vi "face rotate T+.vi"(8 "error in (no error)":errorcluster, 11 "cube in":T1) -> (0 "error out":errorcluster, 3 "cube out":T1)   [LabVIEW 2011]
uses:
  Typedef/cube.ctl
  Typedef/face.ctl
  Typedef/cube rotate direction.ctl
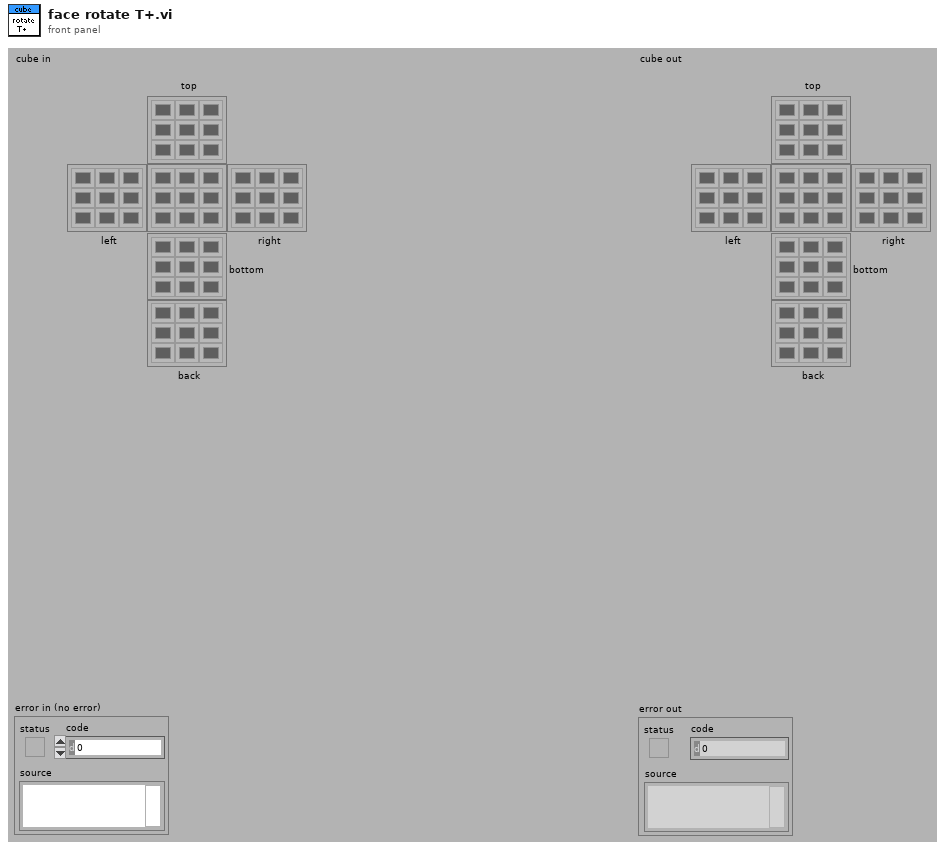
[diagram p1: front panel]
types:
  T1 = typedef "cube.ctl" = cluster{"top":T2, "left":T2, "right":T2, "bottom":T2, "back":T2, "front":T2}
  T2 = typedef "face.ctl" = u32[][]
  T3 = typedef "cube rotate direction.ctl" = enum16{"up", "down", "left", "right"}
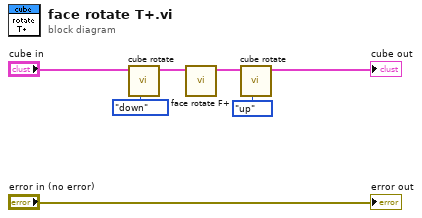
[diagram p0: block diagram]
diagram:
  n1 = call "cube rotate.vi"("cube rotation direction"=cube_rotate_direction."down", "cube in"="cube in") -> ("cube out"=w5:T1)  [unwired: 8 in, 1 out]
  n2 = call "face rotate F+.vi"("cube in"=w5) -> ("cube out"=w3:T1)  [unwired: 9 in, 1 out]
  n3 = call "cube rotate.vi"("cube rotation direction"=cube_rotate_direction."up", "cube in"=w3) -> ("cube out"=→"cube out":T1)  [unwired: 8 in, 1 out]
  "error out" <- "error in (no error)"
